vi "AWGSaveWFFile.vi"() -> ()   [LabVIEW 2017]
uses:
  <vilib>/Utility/file.llb/Write Delimited Spreadsheet (DBL).vi
panel:
  in  "ArbitraryWaveList":dbl[][](array[numeric])=[[100014.0, 200.0, 0.0], [105000.0, 100.0, 0.0], [95000.0, 100.0, 0.0]] caption="Arbitrary Waveform List"
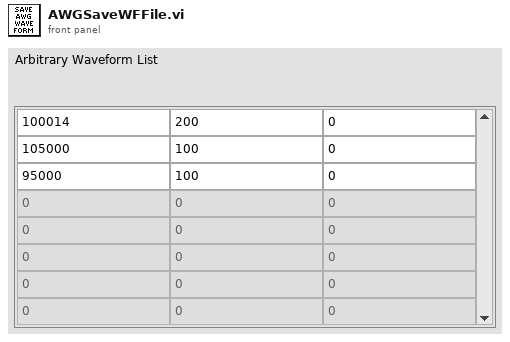
[diagram p1: front panel]
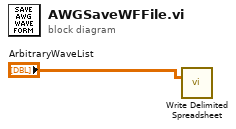
[diagram p0: block diagram]
diagram:
  n1 = call-poly <vilib>:"Write Delimited Spreadsheet.vi"("2D data"="ArbitraryWaveList") -> ()  [unwired: 13 in, 2 out]
